vi "Create Self Enqueuer.vi"(6 "Name":string, 8 "error in (no error)":errorcluster, 11 "VI Refnum":refnum<vi>) -> (0 "error out":errorcluster, 3 "QDMH out":refnum<class "QDMH.lvclass">)   [LabVIEW 2023, in "QDMH.lvlib" / "QDMH.lvclass"]
doc: "This routine uses the Calling VI name to generate unique queue names for self referenced DQMH's or\n\nCreates a named string (if no VI reference provided) that can be called by multiple slave devices."
uses:
  Library/QDMH.lvclass
  Custom Controls/Message.ctl
  Library/QDMH.lvclass/QDMH.ctl
  <vilib>/Utility/error.llb/Trim Whitespace One-Sided.vi
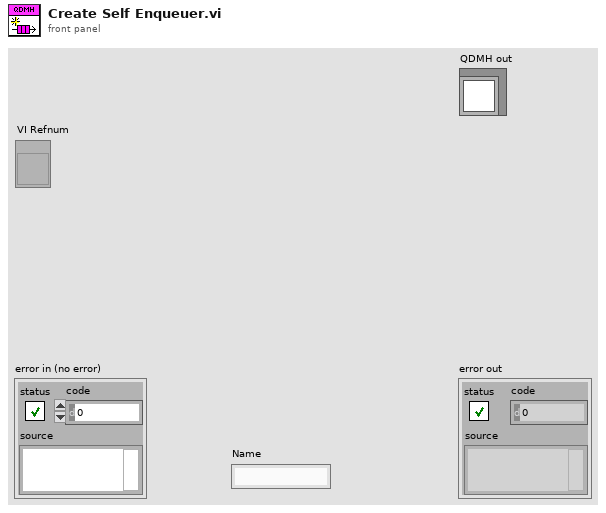
[diagram p1: front panel]
types:
  T1 = typedef "QDMH.lvlib/QDMH.lvclass/Message.ctl" = cluster{"State":string, "Data":variant}
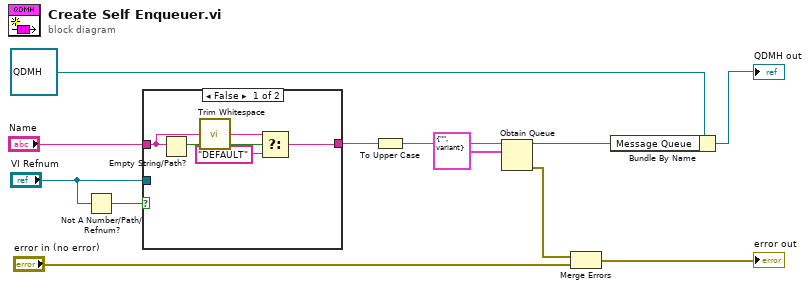
[diagram p0: block diagram]
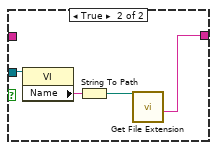
[diagram p2: hidden frame]
diagram:
  n1 = Not A Number/Path/Refnum?(number/path/refnum="VI Refnum") -> (NaN/Path/Refnum?=w11:bool)
  n2 = case shown="False" w11 {
    tunnel: "VI Refnum" -> [_ w21]
    tunnel: "Name" -> [w17 _]
    tunnel: [w14 w18] -> w3
    frame False {
      n3 = Empty String/Path?(string/path=w17) -> (empty?=w16:bool)
      n4 = call <vilib>:"Trim Whitespace.vi"("string"=w17) -> ("trimmed string"=w13:string)  [unwired: 1 in]
      n5 = Select(t=w13, s=w16, f="DEFAULT") -> (s? t:f=w14:string)
    }
    frame True {
      n6 = property class="VI"(reference=w21) -> ("Name"=w19:string)  [unwired: 1 in, 2 out]
      n7 = String To Path(string=w19) -> (path=w20:path)
      n8 = call <vilib>:"Get File Extension.vi"("file"=w20) -> ("filename without extension"=w18:string)  [unwired: 6 in, 4 out]
    }
  }
  n9 = To Upper Case(1:w3) -> (0:w2:string)
  n10 = Obtain Queue(name (unnamed)=w2, element data type=T1 {"State"="", "Data"=variant} ("Message")) -> (queue out=w7:refnum<queue>, error out=w9:errorcluster)  [unwired: 3 in, 1 out]
  n11 = Merge Errors(w9, "error in (no error)") -> (→"error out":errorcluster)
  n12 = Bundle By Name(cluster=refnum<class "QDMH.lvclass"> refnum ("QDMH in"), "Message Queue"=w7) -> (→"QDMH out":refnum<class "QDMH.lvclass">)
